vi "RateControl.vi"(8 "error in (no error)":errorcluster, 11 "Numeric":dbl) -> (0 "error out":errorcluster, 2 "Numeric 3":u32, 3 "Numeric 2":dbl)   [LabVIEW 2021]
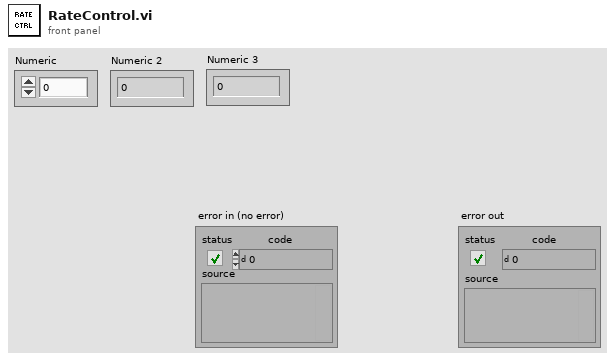
[diagram p1: front panel]
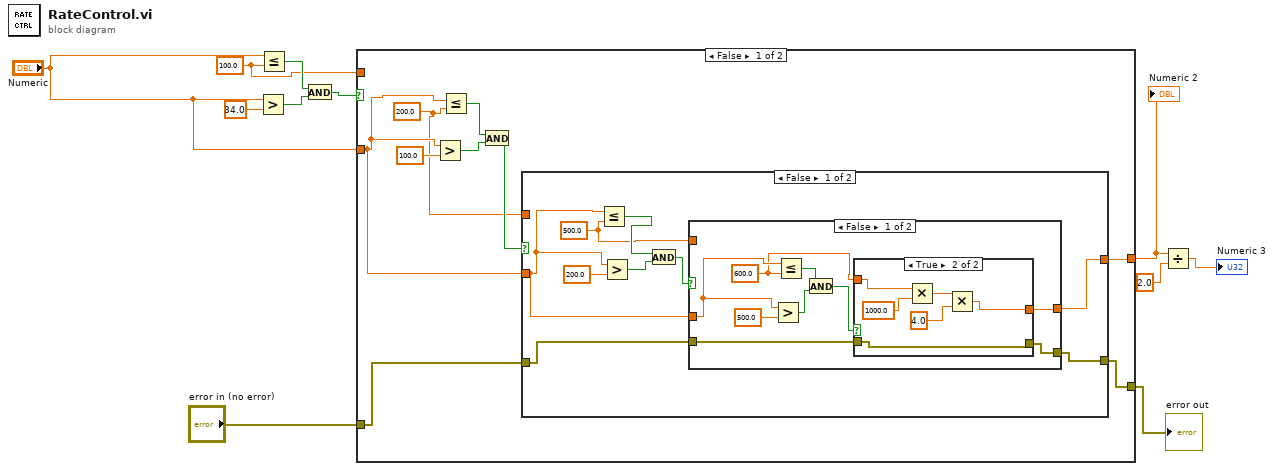
[diagram p0: block diagram]
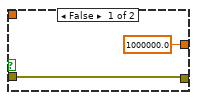
[diagram p2: hidden frame]
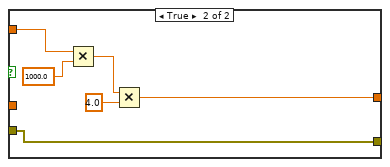
[diagram p3: hidden frame]
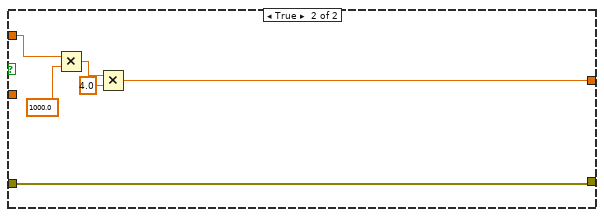
[diagram p4: hidden frame]
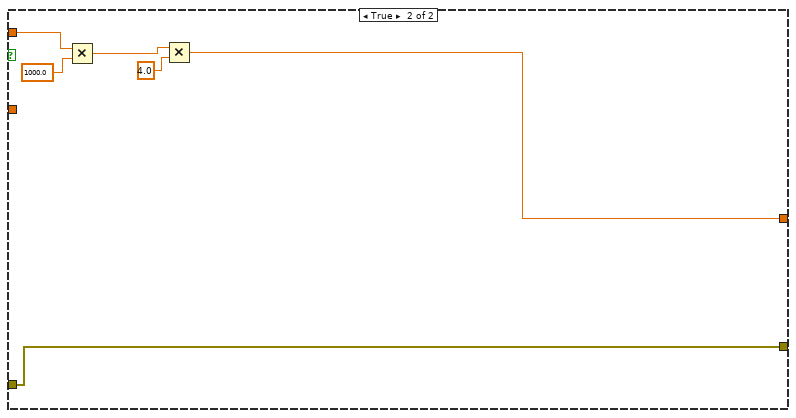
[diagram p5: hidden frame]
diagram:
  w6 = 100.0 ("y")
  n1 = Greater?(x="Numeric", y=34.0) -> (0:w10:bool)
  n2 = Less Or Equal?(x="Numeric", y=w6) -> (x <= y?=w7:bool)
  n3 = And(x=w7, y=w10) -> (x .and. y?=w9:bool)
  n4 = case shown="False" w9 {
    tunnel: [w17 w60] -> w3
    tunnel: w6 -> [_ w62]
    tunnel: "Numeric" -> [w16 _]
    tunnel: "error in (no error)" -> [w13 w59]
    tunnel: [w12 w59] -> w4
    frame False {
      w15 = 200.0 ("y")
      n5 = Greater?(x=w16, y=100.0) -> (0:w19:bool)
      n6 = Less Or Equal?(x=w16, y=w15) -> (x <= y?=w14:bool)
      n7 = And(x=w14, y=w19) -> (x .and. y?=w18:bool)
      n8 = case shown="False" w18 {
        tunnel: [w26 w55] -> w17
        tunnel: w15 -> [_ w54]
        tunnel: w16 -> [w25 _]
        tunnel: w13 -> [w22 w53]
        tunnel: [w21 w53] -> w12
        frame False {
          w23 = 500.0 ("y")
          n9 = Less Or Equal?(x=w25, y=w23) -> (x <= y?=w24:bool)
          n10 = Greater?(x=w25, y=200.0) -> (0:w28:bool)
          n11 = And(x=w24, y=w28) -> (x .and. y?=w27:bool)
          n12 = case shown="False" w27 {
            tunnel: w23 -> [_ w52]
            tunnel: [w35 w49] -> w26
            tunnel: w25 -> [w34 _]
            tunnel: w22 -> [w31 w47]
            tunnel: [w30 w47] -> w21
            frame False {
              w33 = 600.0 ("y")
              n13 = Greater?(x=w34, y=500.0) -> (0:w37:bool)
              n14 = Less Or Equal?(x=w34, y=w33) -> (x <= y?=w32:bool)
              n15 = And(x=w32, y=w37) -> (x .and. y?=w36:bool)
              n16 = case shown="True" w36 {
                tunnel: w33 -> [_ w46]
                tunnel: [1000000.0 w42] -> w35
                tunnel: w31 -> [w39 w41]
                tunnel: [w39 w41] -> w30
                frame False {
                }
                frame True {
                  n17 = Multiply(x=w46, y=1000.0) -> (x*y=w44:dbl)
                  n18 = Multiply(x=w44, y=4.0) -> (x*y=w42:dbl)
                }
              }
            }
            frame True {
              n19 = Multiply(x=w52, y=1000.0) -> (x*y=w51:dbl)
              n20 = Multiply(x=w51, y=4.0) -> (x*y=w49:dbl)
            }
          }
        }
        frame True {
          n21 = Multiply(x=w54, y=1000.0) -> (x*y=w57:dbl)
          n22 = Multiply(x=w57, y=4.0) -> (x*y=w55:dbl)
        }
      }
    }
    frame True {
      n23 = Multiply(x=w62, y=1000.0) -> (x*y=w63:dbl)
      n24 = Multiply(x=w63, y=4.0) -> (x*y=w60:dbl)
    }
  }
  "Numeric 2" <- w3
  "error out" <- w4
  n25 = Divide(x=w3, y=2.0) -> (x/y=→"Numeric 3":dbl)
